vi "OFDM_TransimitPreparation.vi"(10 "IQ rate":dbl, 11 "array":cdb[](array[numeric])) -> (2 "output cluster 2":cluster{"t0":dbl, "dt":dbl, "Y":cdb[]}, 3 "output cluster":cluster{"t0":dbl, "dt":dbl, "Y":cdb[]})   [LabVIEW 2018]
panel:
  out "size(s)":i32
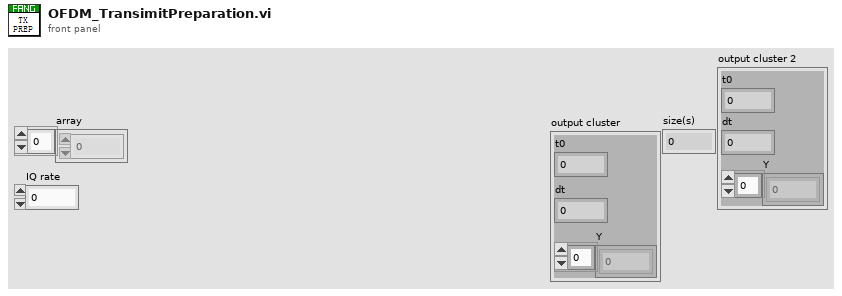
[diagram p1: front panel]
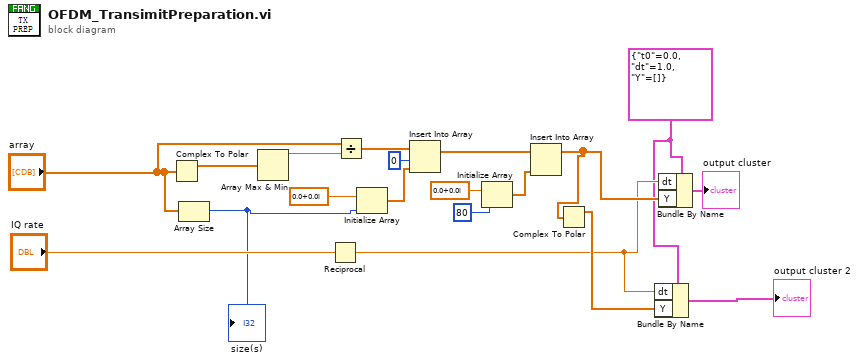
[diagram p0: block diagram]
diagram:
  w1 = cluster{"t0":dbl, "dt":dbl, "Y":cdb[]} {"t0"=0.0, "dt"=1.0, "Y"=[]} ("data")
  n1 = Complex To Polar(r * e^(i*theta)="array") -> (r=w19:dbl[])  [unwired: 1 out]
  n2 = Array Size(array="array") -> (size(s)=w6:i32)
  "size(s)" <- w6
  n3 = Array Max & Min(array=w19) -> (max value=w18:dbl)  [unwired: 3 out]
  n4 = Reciprocal(x="IQ rate") -> (1/x=w3:dbl)
  n5 = Divide(x="array", y=w18) -> (x/y=w17:cdb[])
  n6 = Initialize Array(cdb 0.0+0.0i ("element"), w6) -> (w13:cdb[])
  n7 = Insert Into Array(array=w17, index=0, new element=w13) -> (w14:cdb[])
  n8 = Initialize Array(cdb 0.0+0.0i ("element"), 80 ("dimension size")) -> (w11:cdb[])
  n9 = Insert Into Array(array=w14, new element=w11) -> (w5:cdb[])  [unwired: 1 in]
  n10 = Complex To Polar(r * e^(i*theta)=w5) -> (r=w4:dbl[])  [unwired: 1 out]
  n11 = Bundle By Name(cluster=w1, "dt"=w3, "Y"=w4) -> (→"output cluster 2":cluster{"t0":dbl, "dt":dbl, "Y":cdb[]})
  n12 = Bundle By Name(cluster=w1, "dt"=w3, "Y"=w5) -> (→"output cluster":cluster{"t0":dbl, "dt":dbl, "Y":cdb[]})
